vi "Check Query Options.vi"(8 "error in (no error)":errorcluster, 11 "TCP Client in":refnum<class "TCP Client.lvclass">) -> (0 "error out":errorcluster, 3 "TCP Client out":refnum<class "TCP Client.lvclass">)   [LabVIEW 2012, in "Stream-TCP.lvlib" / "TCP Client.lvclass"]
uses:
  TCP Client.lvclass
  lv-stream/stream/Endpoint/Endpoint.lvclass
  lv-stream/stream/URI/URI.lvclass
  TCP Mode.ctl
  Stream-TCP.lvlib
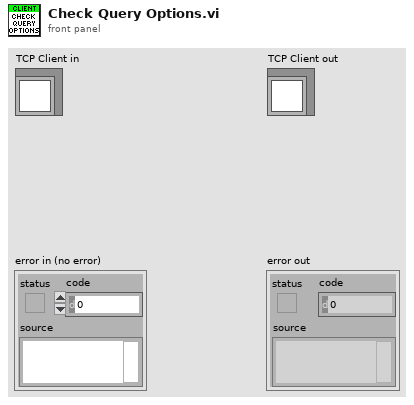
[diagram p1: front panel]
types:
  T1 = typedef "Stream-TCP.lvlib/TCP Mode.ctl" = enum16{"buffered", "raw"}
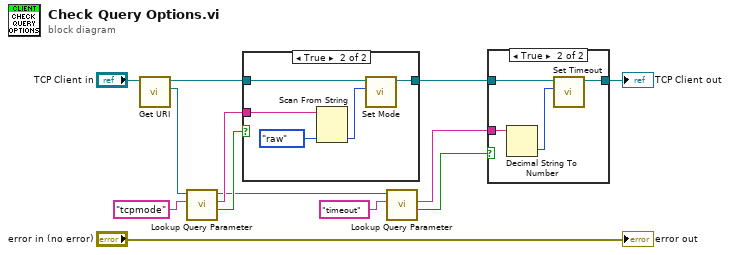
[diagram p0: block diagram]
diagram:
  n1 = call "Get URI.vi"("Endpoint in"="TCP Client in") -> ("URI"=w11:refnum<class "URI.lvclass">, "Endpoint out"=w7:refnum<class "TCP Client.lvclass">)  [unwired: 8 in, 1 out]
  n2 = call "Lookup Query Parameter.vi"("Name"="tcpmode", "URI in"=w11) -> ("Found"=w9:bool, "Value"=w8:string, "URI out"=w5:refnum<class "URI.lvclass">)  [unwired: 6 in, 1 out]
  n3 = case shown="True" w9 {
    tunnel: w8 -> [_ w19]
    tunnel: w7 -> [w14 w17]
    tunnel: [w14 w15] -> w4
    frame False {
    }
    frame True {
      n4 = Scan From String(input string=w19, default 1=TCP_Mode."raw" ("TCP Mode")) -> (output 1=w16:T1)  [unwired: 3 in, 3 out]
      n5 = call "Set Mode.vi"("TCP Mode"=w16, "TCP Client in"=w17) -> ("TCP Client out"=w15:refnum<class "TCP Client.lvclass">)  [unwired: 8 in, 1 out]
    }
  }
  n6 = call "Lookup Query Parameter.vi"("Name"="timeout", "URI in"=w5) -> ("Found"=w3:bool, "Value"=w2:string)  [unwired: 6 in, 2 out]
  n7 = case shown="True" w3 {
    tunnel: w4 -> [w20 w23]
    tunnel: w2 -> [_ w24]
    tunnel: [w20 w21] -> w1
    frame False {
    }
    frame True {
      n8 = Decimal String To Number(string=w24) -> (number=w22:i32)  [unwired: 2 in, 1 out]
      n9 = call "Set Timeout.vi"("Timeout ms"=w22, "TCP Client in"=w23) -> ("TCP Client out"=w21:refnum<class "TCP Client.lvclass">)  [unwired: 8 in, 1 out]
    }
  }
  "TCP Client out" <- w1
  "error out" <- "error in (no error)"
